vi "文件路径.vi"(1 "文件名":string) -> (0 "数组":path[](array[path]))   [LabVIEW 2012]
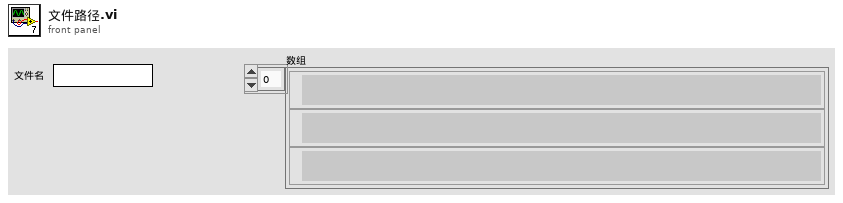
[diagram p1: front panel]
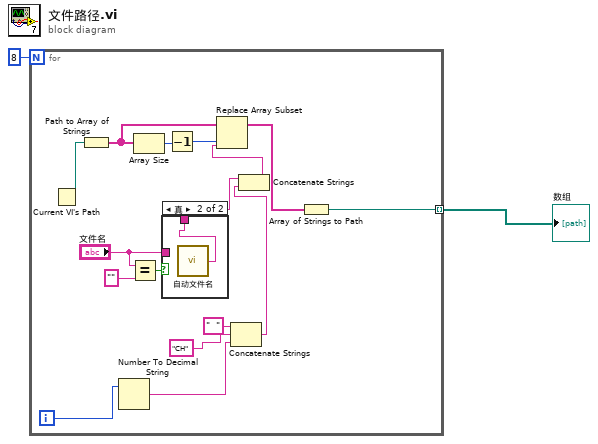
[diagram p0: block diagram]
diagram:
  n1 = for {
    N: 8 -> [_]
    tunnel: [w11] -> w1 mode=indexing
    i -> [w10]
    n2 = Current VI's Path() -> (path=w18:path)
    n3 = Path to Array of Strings ("路径至字符串数组转换")(0:w18) -> (2:w17:string[])  [unwired: 1 out]
    n4 = Number To Decimal String(number=w10) -> (decimal integer string=w7:string)  [unwired: 1 in]
    n5 = Equal?(x="文件名", y="") -> (x = y?=w13:bool)
    n6 = Array Size(array=w17) -> (size(s)=w16:i32)
    n7 = case shown="真" w13 {
      tunnel: "文件名" -> [w19 _]
      tunnel: [w19 w20] -> w6
      frame False {
      }
      frame True {
        n8 = call "自动文件名.vi"() -> ("日期/时间字符串"=w20:string)
      }
    }
    n9 = Decrement(x=w16) -> (x-1=w15:i32)
    n10 = Concatenate Strings("  " ("字符串"), "CH" ("元素"), w7) -> (w5:string)
    n11 = Concatenate Strings(w6, w5) -> (w4:string)
    n12 = Replace Array Subset(array=w17, new element=w4, index=w15) -> (w9:string[])
    n13 = Array of Strings to Path(0:w9) -> (2:w11:path)  [unwired: 1 in]
  }
  "数组" <- w1
